vi "Decompress Message Data.vi"(10 "Compression (zip)":T1, 11 "Compressed Message":u8[](array[numeric])) -> (3 "Message":string)   [LabVIEW 2020]
uses:
  Compression Type.ctl
  <vilib>/zip/NI_Unzip.lvlib
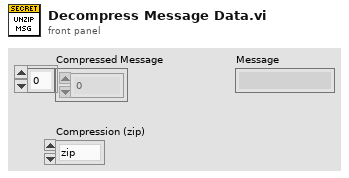
[diagram p1: front panel]
types:
  T1 = typedef "Compression Type.ctl" = enum16{"zip", "7z"}
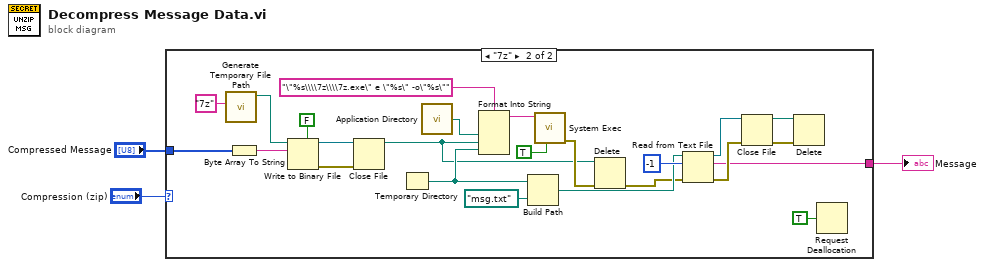
[diagram p0: block diagram]
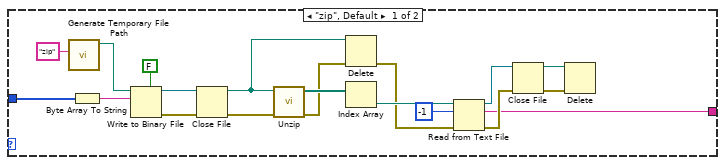
[diagram p2: hidden frame]
diagram:
  n1 = case shown="\"7z\"" "Compression (zip)" {
    tunnel: "Compressed Message" -> [w7 w37]
    tunnel: [w5 w35] -> w2
    frame "zip", Default {
      n2 = call <vilib>:"Generate Temporary File Path.vi"("Temporary File Extension (tmp)"="zip") -> ("Unique Temporary File Path"=w13:path)  [unwired: 9 in, 1 out]
      n3 = Byte Array To String(unsigned byte array=w7) -> (string=w6:string)
      n4 = Write to Binary File(file (use dialog)=w13, data=w6, 5:FALSE ("prepend array or string size? (T)")) -> (refnum out=w22:refnum<file>, error out=w12:errorcluster)  [unwired: 3 in, 1 out]
      n5 = Close File(refnum=w22, error in=w12) -> (path=w16:path, error out=w11:errorcluster)
      n6 = call <vilib>:"Unzip.vi"("error in (no error)"=w11, "Zip file"=w16) -> ("error out"=w15:errorcluster, "Unzipped files"=w21:path[])  [unwired: 7 in, 1 out]
      n7 = Delete(path (use dialog)=w16, error in=w15) -> (error out=w10:errorcluster)  [unwired: 3 in, 2 out]
      n8 = Index Array(array=w21) -> (element=w20:path)  [unwired: 1 in]
      n9 = Read from Text File(file (use dialog)=w20, count=-1, error in=w10) -> (refnum out=w18:refnum<file>, text=w5:string, error out=w9:errorcluster)  [unwired: 1 in, 1 out]
      n10 = Close File(refnum=w18, error in=w9) -> (path=w17:path, error out=w8:errorcluster)
      n11 = Delete(path (use dialog)=w17, error in=w8) -> ()  [unwired: 3 in, 3 out]
    }
    frame "7z" {
      n12 = call <vilib>:"Generate Temporary File Path.vi"("Temporary File Extension (tmp)"="7z") -> ("Unique Temporary File Path"=w41:path)  [unwired: 9 in, 1 out]
      n13 = Byte Array To String(unsigned byte array=w37) -> (string=w36:string)
      n14 = Write to Binary File(file (use dialog)=w41, data=w36, 5:FALSE ("prepend array or string size? (T)")) -> (refnum out=w46:refnum<file>, error out=w40:errorcluster)  [unwired: 3 in, 1 out]
      n15 = Close File(refnum=w46, error in=w40) -> (path=w26:path)  [unwired: 1 out]
      n16 = Temporary Directory() -> (w32:path)
      n17 = call <vilib>:"Application Directory.vi"() -> ("Application Directory"=w29:path)
      n18 = Format Into String(format string="\"%s\\\\7z\\\\7z.exe\" e \"%s\" -o\"%s\"" ("command line"), w29, w26, w32) -> (resulting string=w33:string)  [unwired: 2 in, 1 out]
      n19 = Build Path(base path=w32, name or relative path=path "msg.txt") -> (appended path=w30:path)
      n20 = call <vilib>:"System Exec.vi"("run minimized? (F)"=TRUE, "command line"=w33) -> ("error out"=w27:errorcluster)  [unwired: 6 in, 3 out]
      n21 = Delete(path (use dialog)=w26, error in=w27) -> (error out=w25:errorcluster)  [unwired: 3 in, 2 out]
      n22 = Read from Text File(file (use dialog)=w30, count=-1, error in=w25) -> (refnum out=w44:refnum<file>, text=w35:string, error out=w39:errorcluster)  [unwired: 1 in, 1 out]
      n23 = Close File(refnum=w44, error in=w39) -> (path=w43:path, error out=w38:errorcluster)
      n24 = Delete(path (use dialog)=w43, error in=w38) -> ()  [unwired: 3 in, 3 out]
      n25 = Request Deallocation(TRUE ("flag")) -> ()
    }
  }
  "Message" <- w2
